vi "pose_to_vector.vi"(4 "Angle unit":enum16{"Radians", "Degrees"}(ring)=enum."Degrees", 6 "Translation scale":dbl=0.001 format="%#_6p", 11 "Pose":T1=[[1.0, 0.0, 0.0, 0.0], [0.0, 1.0, 0.0, 0.0], [0.0, 0.0, 1.0, 0.0], [0.0, 0.0, 0.0, 1.0]]) -> (3 "Pose vector":dbl[](array[numeric]))   [LabVIEW 2013]
uses:
  <vilib>/Analysis/Matrix/Datatypes/RealMatrix.ctl
  <vilib>/Analysis/coordinate.llb/Angle Units.ctl
  <vilib>/Analysis/coordinate.llb/Euler Rotation Order.ctl
  <vilib>/Analysis/coordinate.llb/Wrap Angle (scalar).vi
  <vilib>/Analysis/NI_AAL_Angle.lvlib
  <vilib>/Analysis/NI_AALPro.lvlib
  <vilib>/Analysis/Matrix/NI_Matrix.lvlib
panel:
  # "Convert a pose to a vector using Euler angle representation.   X Y Z Rx Ry Rz"
  # "Multiply XYZ by this."
  # "Rotations in degrees or radians?"
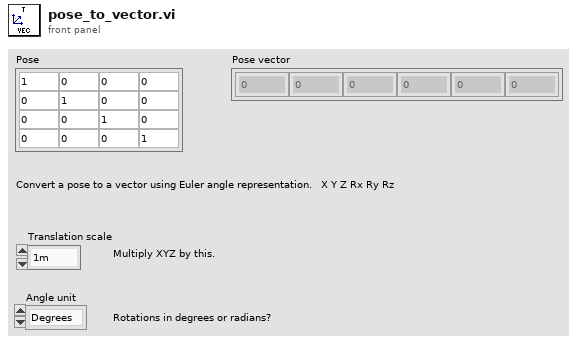
[diagram p1: front panel]
types:
  T1 = typedef "NI_Matrix.lvlib/RealMatrix.ctl" = dbl[][]
  T2 = typedef "NI_AALPro.lvlib/Euler Rotation Order.ctl" = u16
  T3 = typedef "NI_AAL_Angle.lvlib/Angle Units.ctl" = i32
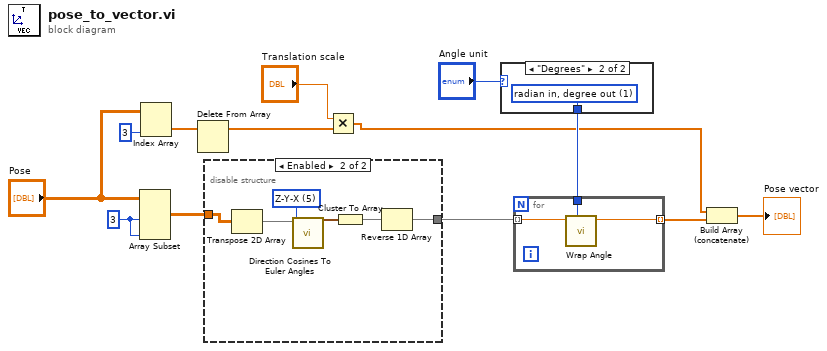
[diagram p0: block diagram]
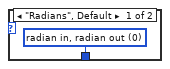
[diagram p2: hidden frame]
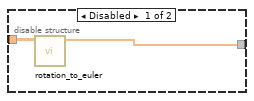
[diagram p3: hidden frame]
diagram:
  w10 = 3 ("length")
  n1 = Array Subset(array="Pose", length (row)=w10, length (col)=w10) -> (w11:T1)  [unwired: 2 in]
  n2 = Index Array(array="Pose", index (col)=3 ("disabled index (col)")) -> (element=w7:dbl[])  [unwired: 1 in]
  n3 = Delete From Array(array=w7) -> (array with subset deleted=w3:dbl[])  [unwired: 2 in, 1 out]
  n4 = disable-structure shown="Enabled" {
    disable-tunnel: [w15 w18] -> w6
    disable-tunnel: w11 -> [w14 w17]
    frame Disabled {
      n5 = call "rotation_to_euler.vi"("Rotation"=w14) -> ("Theta XYZ"=w15:dbl[])  [unwired: 10 in]
    }
    frame Enabled {
      w20 = T2 5 items=["X-Y-Z", "X-Z-Y", "Y-X-Z", "Y-Z-X", "Z-X-Y", "Z-Y-X", "X-Y-X", "X-Z-X", "Y-X-Y", "Y-Z-Y", "Z-X-Z", "Z-Y-Z"] ("rotation order")
      n6 = Transpose 2D Array(2D array=w17) -> (transposed array=w16:T1)
      n7 = call <vilib>:"Direction Cosines To Euler Angles.vi"("rotation order"=w20, "Direction Cosines"=w16) -> ("Euler Angles"=w21:cluster{"phi":dbl, "theta":dbl, "psi":dbl})  [unwired: 8 in, 1 out]
      n8 = Cluster To Array(cluster=w21) -> (array=w19:dbl[])
      n9 = Reverse 1D Array(array=w19) -> (reversed array=w18:dbl[])
    }
  }
  n10 = Multiply(x="Translation scale", y=w3) -> (x*y=w2:dbl[])
  n11 = case shown="\"Degrees\"" "Angle unit" {
    tunnel: [w22 w23] -> w4
    frame "Radians", Default {
      w22 = T3 0 items=["radian in, radian out", "radian in, degree out", "degree in, degree out", "degree in, radian out"] ("angle units")
    }
    frame "Degrees" {
      w23 = T3 1 items=["radian in, radian out", "radian in, degree out", "degree in, degree out", "degree in, radian out"] ("angle units")
    }
  }
  n12 = for {
    tunnel: w6 -> [w26] mode=indexing
    tunnel: [w25] -> w9 mode=indexing
    tunnel: w4 -> [w24]
    n13 = call-poly <vilib>:"Wrap Angle.vi"("angle units"=w24, "angle in"=w26) -> ("angle out"=w25:dbl)  [unwired: 8 in, 1 out]
  }
  n14 = Build Array (concatenate)(w2, w9) -> (→"Pose vector":dbl[])
